vi "parts.set.vi"(8 "error in (no error)":errorcluster, 10 "Parts":T1(array[cluster]), 11 "Multipart Upload in":refnum<class "Multipart Upload.lvclass">) -> (0 "error out":errorcluster, 3 "Multipart Upload out":refnum<class "Multipart Upload.lvclass">)   [LabVIEW 2020, in "Multipart Upload.lvclass"]
uses:
  Multipart Upload.lvclass
  Multipart Upload.lvclass/Multipart Upload.ctl
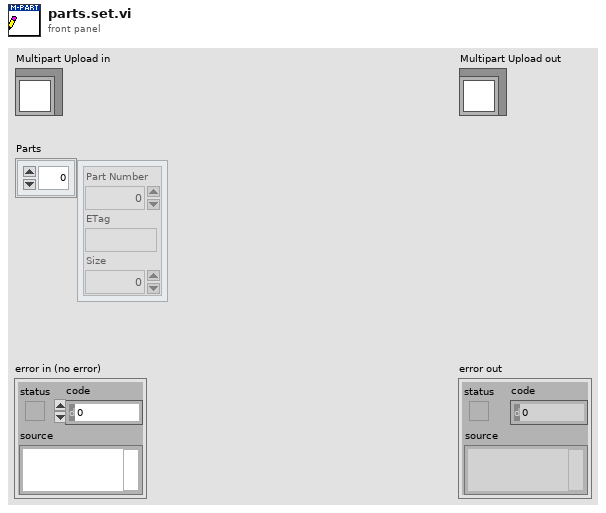
[diagram p1: front panel]
types:
  T1 = cluster{"Part Number":i32, "ETag":string, "Size":i32}[]
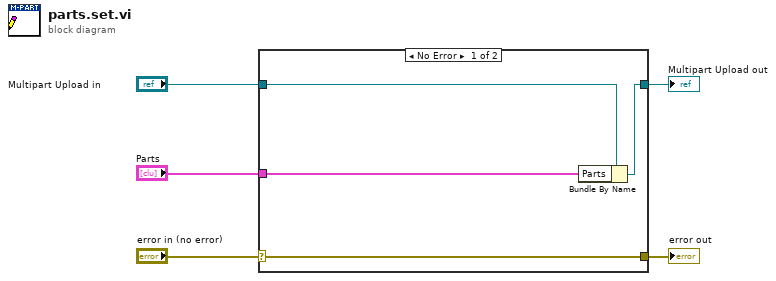
[diagram p0: block diagram]
diagram:
  n1 = case shown="No Error" "error in (no error)" {
    selector: "error in (no error)" -> [w9 w10]
    tunnel: [w9 w10] -> w4
    tunnel: [w7 w11] -> w2
    tunnel: "Multipart Upload in" -> [w8 w11]
    tunnel: "Parts" -> [w6 _]
    frame No Error {
      n2 = Bundle By Name(cluster=w8, "Parts"=w6) -> (w7:refnum<class "Multipart Upload.lvclass">)
    }
    frame Error {
    }
  }
  "error out" <- w4
  "Multipart Upload out" <- w2
